vi "CallPython_AssertExpectedResult.vi"() -> ()   [LabVIEW 2013]
uses:
  PythonTools.lvclass
  <vilib>/addons/_JKI Toolkits/Caraya/classes/Test/Test.lvclass
  <vilib>/addons/_JKI Toolkits/Caraya/classes/Assert/Assert.lvclass
panel:
  in  "error in (no error)":errorcluster
  out "error out":errorcluster
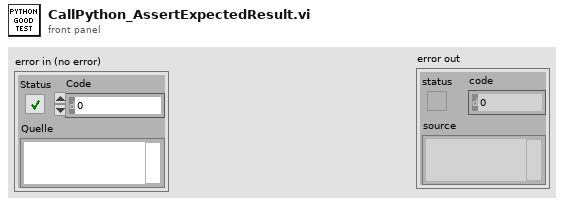
[diagram p1: front panel]
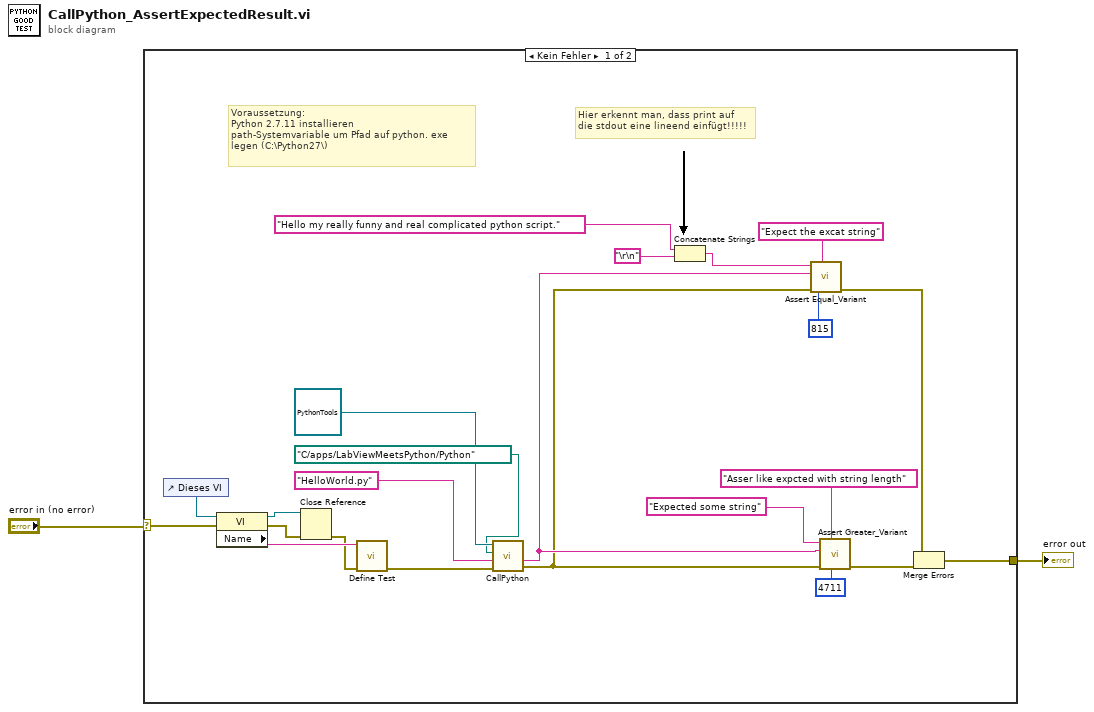
[diagram p0: block diagram]
diagram:
  n1 = case shown="Kein Fehler" "error in (no error)" {
    selector: "error in (no error)" -> [w23 w26]
    tunnel: [w19 w26] -> w2
    frame No Error {
      # "Voraussetzung:\nPython 2.7.11 installieren\npath-Systemvariable um Pfad auf python. exe \nlegen (C:\\Python27\\)"
      # "Hier erkennt man, dass print auf\ndie stdout eine lineend einfügt!!!!!"
      n2 = control-ref of="Dieses VI"() -> (w25:refnum<vi>)
      n3 = property class="VI"(reference=w25, error in=w23) -> (reference out=w22:refnum<vi>, error out=w21:errorcluster, "Name"=w24:string)
      n4 = Close Reference(reference=w22, error in (no error)=w21) -> (error out=w20:errorcluster)
      n5 = call <vilib>:"Define Test.vi"("error in (no error)"=w20, "Label (VI Title)"=w24) -> ("error out"=w17:errorcluster)  [unwired: 9 in]
      n6 = call "CallPython.vi"("error in (no error)"=w17, "command line"="HelloWorld.py", "working directory"=path "C:/apps/LabViewMeetsPython/Python", "PythonTools.lvclass"=refnum<class "PythonTools.lvclass"> refnum) -> ("error out"=w9:errorcluster, "standard output"=w10:string)  [unwired: 4 in, 2 out]
      n7 = Concatenate Strings("Hello my really funny and real complicated python script." ("Label"), "\r\n") -> (w3:string)
      n8 = call <vilib>:"Assert Equal_Variant.vi"("error code (1)"=815, "Label"="Expect the excat string", "error in (no error)"=w9, "Y"=w10, "X"=w3) -> ("error out"=w8:errorcluster)  [unwired: 6 in]
      n9 = call <vilib>:"Assert Greater_Variant.vi"("error code (1)"=4711, "Label"="Asser like expcted with string length", "error in (no error)"=w9, "Y"=w10, "X"="Expected some string" ("Label")) -> ("error out"=w13:errorcluster)  [unwired: 6 in]
      n10 = Merge Errors(w8, w13) -> (w19:errorcluster)
    }
    frame Error {
    }
  }
  "error out" <- w2
